vi "Read Control Name.vi"(8 "error in (no error)":errorcluster, 11 "Control Info in":refnum<class "Control Info.lvclass">) -> (0 "error out":errorcluster, 2 "Control Name":string, 3 "Control Info out":refnum<class "Control Info.lvclass">)   [LabVIEW 2017, in "Localization.lvlib" / "Control Info.lvclass"]
doc: "Read the Control Name from the class data.\n\nChoose Movement Consulting, LLC"
uses:
  Control Info.lvclass
  Control Info.lvclass/Control Info.ctl
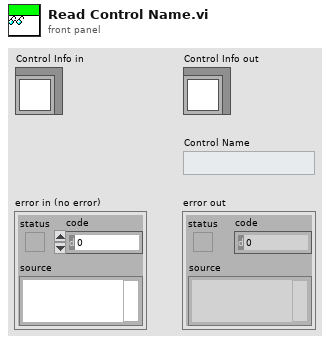
[diagram p1: front panel]
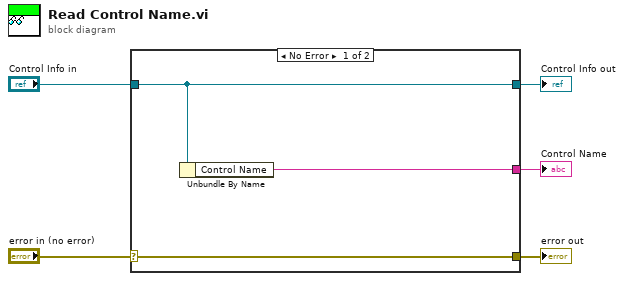
[diagram p0: block diagram]
diagram:
  n1 = case shown="No Error" "error in (no error)" {
    selector: "error in (no error)" -> [w8 w9]
    tunnel: [w8 w9] -> w4
    tunnel: [w7 w10] -> w2
    tunnel: "Control Info in" -> [w7 w10]
    tunnel: [w6 _] -> w1
    frame No Error {
      n2 = Unbundle By Name(w7) -> ("Control Name"=w6:string)
    }
    frame Error {
    }
  }
  "error out" <- w4
  "Control Info out" <- w2
  "Control Name" <- w1
